vi "Destroy.vi"(8 "error in (no error)":errorcluster, 11 "Conditional in":refnum<class "Conditional.lvclass">) -> (0 "error out":errorcluster)   [LabVIEW 2017, in "Test Executive.lvlib" / "Conditional.lvclass"]
uses:
  <vilib>/gpm_packages/@cs/test-executive/Source/Test Executive/Conditional/Conditional.lvclass
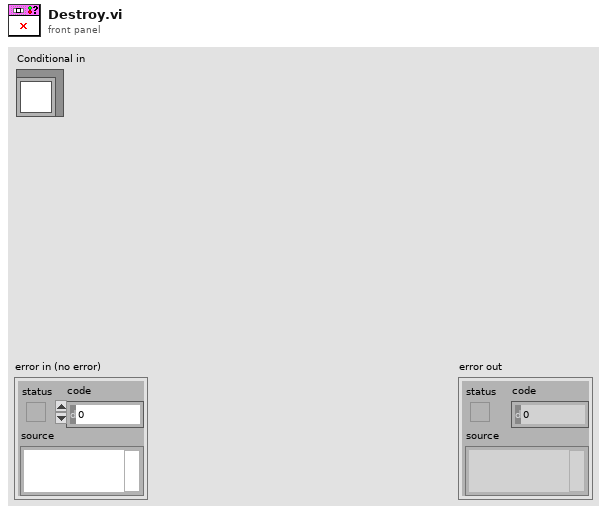
[diagram p1: front panel]
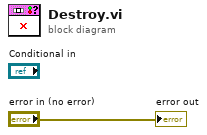
[diagram p0: block diagram]
diagram:
  "error out" <- "error in (no error)"
